vi "Configure Trigger.vi"(6 "Trigger Delay (0.1 s)":dbl=0.1 min=0.1 max=9999.9 step=1.0 format="%.1f", 7 "Channel (1:1)":u16(ring)=1 items=["1"=1, "2"=2, "3"=3], 8 "error in (no error)":errorcluster, 9 "Triggered Current Limit (0.0 A)":dbl min=0.0 max=25.0 step=1.0 format="%.3f", 10 "Triggered Voltage Level (0.000 V)":dbl min=0.0 max=61.0 step=0.001 format="%.3f", 11 "VISA resource name":refnum<visa-resource-name>) -> (0 "error out":errorcluster, 3 "VISA resource name out":refnum<visa-resource-name>)   [LabVIEW 2017, in "BK Precision 913XX.lvlib"]
doc: "Configures the triggered voltage level, current limit, and trigger delay. When triggered, the instrument will set to the configured trigger values."
uses:
  <instrlib>/BK Precision 913XX/BK Precision 913XX.lvlib
panel:
  # "V"
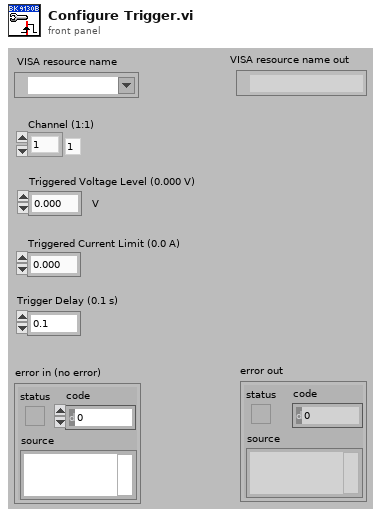
[diagram p1: front panel]
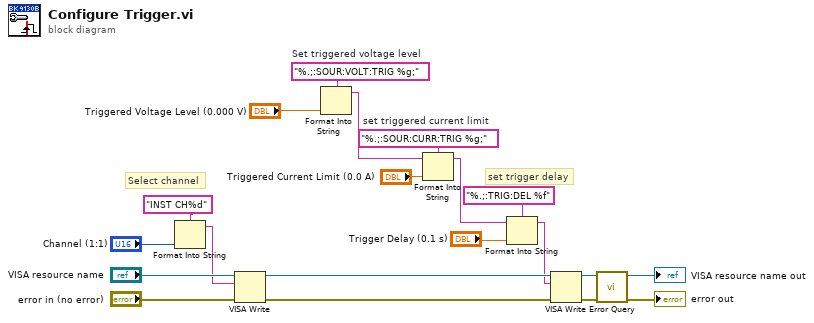
[diagram p0: block diagram]
diagram:
  w7 = "%.;:SOUR:CURR:TRIG %g;"  # set triggered current limit
  w16 = "%.;:SOUR:VOLT:TRIG %g;"  # Set triggered voltage level
  # "set trigger delay"
  # "Select channel"
  n1 = Format Into String(format string="INST CH%d", "Channel (1:1)") -> (resulting string=w9:string)  [unwired: 2 in, 1 out]
  n2 = VISA Write(VISA resource name="VISA resource name", write buffer=w9, error in (no error)="error in (no error)") -> (VISA resource name out=w11:refnum<visa-resource-name>, error out=w12:errorcluster)  [unwired: 1 out]
  n3 = Format Into String(format string=w16, "Triggered Voltage Level (0.000 V)") -> (resulting string=w5:string)  [unwired: 2 in, 1 out]
  n4 = Format Into String(format string=w7, initial string=w5, "Triggered Current Limit (0.0 A)") -> (resulting string=w3:string)  [unwired: 1 in, 1 out]
  n5 = Format Into String(format string="%.;:TRIG:DEL %f", initial string=w3, "Trigger Delay (0.1 s)") -> (resulting string=w1:string)  [unwired: 1 in, 1 out]
  n6 = VISA Write(VISA resource name=w11, write buffer=w1, error in (no error)=w12) -> (VISA resource name out=w17:refnum<visa-resource-name>, error out=w18:errorcluster)  [unwired: 1 out]
  n7 = call <instrlib>:"Error Query.vi"("error in (no error)"=w18, "VISA resource name"=w17) -> ("error out"=→"error out":errorcluster, "VISA resource name out"=→"VISA resource name out":refnum<visa-resource-name>)  [unwired: 6 in, 2 out]
